vi "insertion sorting.vi"(11 "input":dbl[](array[numeric])) -> (3 "sorted":dbl[](array[numeric]))   [LabVIEW 2014]
panel:
  out "temp":dbl[](array[numeric])
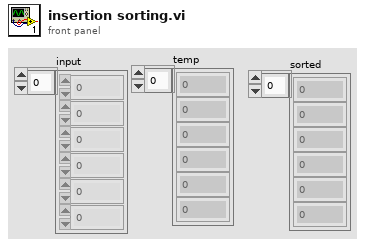
[diagram p1: front panel]
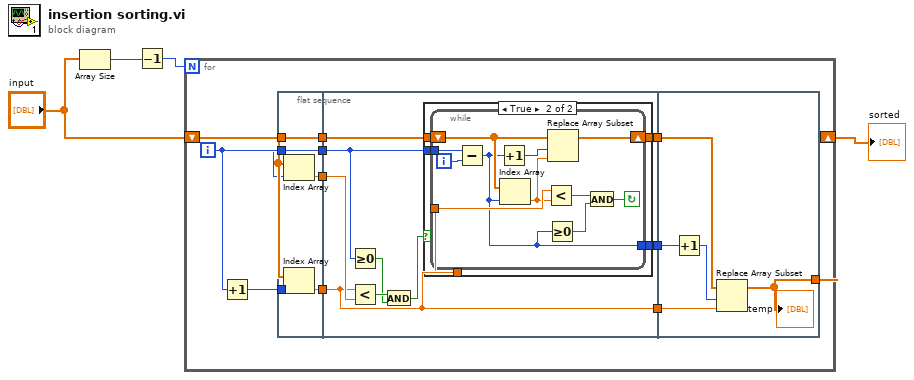
[diagram p0: block diagram]
diagram:
  n1 = Array Size(array="input") -> (size(s)=w3:i32)
  n2 = Decrement(x=w3) -> (x-1=w4:i32)
  n3 = for {
    N: w4 -> [_]
    shift-right: [w5] -> w2
    shift-left: "input" -> [w13]
    i -> [w14]
    n4 = Increment(x=w14) -> (x+1=w15:i32)
    n5 = flat-sequence {
      tunnel: w15 -> [w17]
      tunnel: w14 -> [w16]
      tunnel: w13 -> [w18]
      tunnel: [w20] -> w12
      tunnel: [w19] -> w11
      tunnel: [w18] -> w10
      tunnel: [w16] -> w9
      tunnel: w12 -> [w25]
      tunnel: w11 -> [w21]
      tunnel: w10 -> [w26]
      tunnel: w9 -> [w24]
      tunnel: [w23] -> w8
      tunnel: [w22] -> w7
      tunnel: [w21] -> w6
      tunnel: w8 -> [w50]
      tunnel: w7 -> [w51]
      tunnel: w6 -> [w49]
      tunnel: [w48] -> w5
      frame #0 {
        n6 = Index Array(array=w18, index=w16) -> (element=w20:dbl)
        n7 = Index Array(array=w18, index=w17) -> (element=w19:dbl)
      }
      frame #1 {
        n8 = Greater Or Equal To 0?(x=w24) -> (x >= 0?=w28:bool)
        n9 = Less?(x=w21, y=w25) -> (x < y?=w29:bool)
        n10 = And(x=w29, y=w28) -> (x .and. y?=w27:bool)
        n11 = case shown="True" w27 {
          tunnel: w24 -> [w31 w36]
          tunnel: w26 -> [w30 w35]
          tunnel: w21 -> [_ w34]
          tunnel: [w31 w33] -> w23
          tunnel: [w30 w32] -> w22
          frame False {
          }
          frame True {
            n12 = while {
              shift-right: [w43] -> w32
              shift-left: w35 -> [w44]
              tunnel: w36 -> [w47]
              tunnel: w34 -> [w42]
              tunnel: [w37] -> w33
              i -> [w46]
              stop <- w38 continue-if-true
              n13 = Subtract(x=w47, y=w46) -> (x-y=w37:i32)
              n14 = Increment(x=w37) -> (x+1=w45:i32)
              n15 = Index Array(array=w44, index=w37) -> (element=w41:dbl)
              n16 = Less?(x=w42, y=w41) -> (x < y?=w40:bool)
              n17 = Greater Or Equal To 0?(x=w37) -> (x >= 0?=w39:bool)
              n18 = Replace Array Subset(array=w44, new element=w41, index=w45) -> (w43:dbl[])
              n19 = And(x=w40, y=w39) -> (x .and. y?=w38:bool)
            }
          }
        }
      }
      frame #2 {
        n20 = Increment(x=w50) -> (x+1=w52:i32)
        n21 = Replace Array Subset(array=w51, new element=w49, index=w52) -> (w48:dbl[])
        "temp" <- w48
      }
    }
  }
  "sorted" <- w2
